vi "Save Symbol.vi"(8 "error in (no error)":errorcluster, 10 "path":path, 11 "proj ref":refnum<vi>) -> (0 "error out":errorcluster, 2 "path out":path, 3 "proj ref out":refnum<vi>)   [LabVIEW 2014, in "lvprj2html.lvlib"]
uses:
  lvprj2html.lvlib
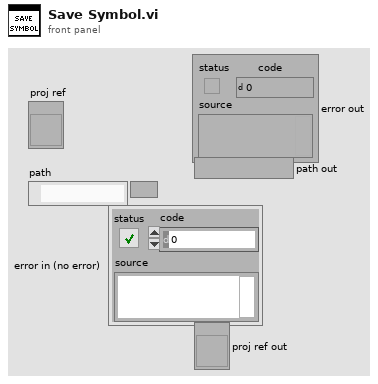
[diagram p1: front panel]
types:
  T1 = typedef "imagedata.ctl" = cluster{"image type":i32, "image depth":i32, "image":u8[], "mask":u8[], "colors":u32[], "Rectangle":cluster{"left":i16, "top":i16, "right":i16, "bottom":i16}}
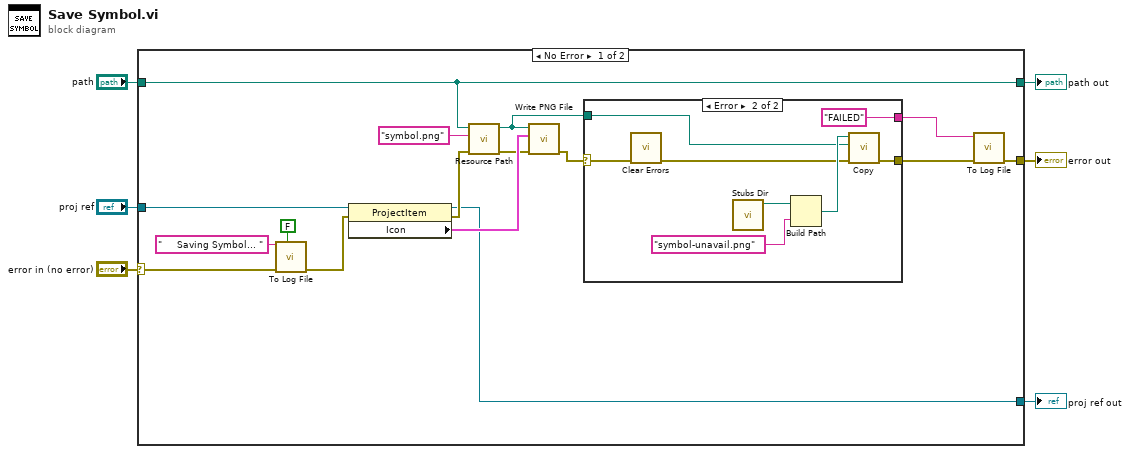
[diagram p0: block diagram]
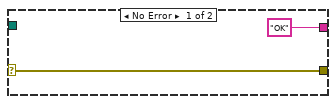
[diagram p2: hidden frame]
diagram:
  n1 = case shown="No Error" "error in (no error)" {
    selector: "error in (no error)" -> [w8 w35]
    tunnel: "proj ref" -> [w21 w33]
    tunnel: [w17 w33] -> w5
    tunnel: "path" -> [w7 w34]
    tunnel: [w9 w35] -> w3
    tunnel: [w7 w34] -> w1
    frame No Error {
      n2 = call "To Log File.vi"("new line"=FALSE, "error in (no error)"=w8, "string"="     Saving Symbol... " ("format string")) -> ("error out"=w14:errorcluster)  [unwired: 8 in]
      n3 = property class="ProjectItem"(reference=w21, error in=w14) -> (reference out=w17:refnum<vi>, error out=w19:errorcluster, "Icon"=w22:T1)
      n4 = call "Resource Path.vi"("error in (no error)"=w19, "resource file name"="symbol.png", "data dir"=w7) -> ("error out"=w18:errorcluster, "path"=w11:path)  [unwired: 7 in]
      n5 = call <vilib>:"Write PNG File.vi"("error in (no error)"=w18, "image data"=w22, "path to PNG file"=w11) -> ("error out"=w10:errorcluster)  [unwired: 7 in, 1 out]
      n6 = case shown="Error" w10 {
        selector: w10 -> [w24 w32]
        tunnel: [w24 w25] -> w12
        tunnel: ["OK" ("string") "FAILED" ("string")] -> w13
        tunnel: w11 -> [_ w27]
        frame No Error {
        }
        frame Error {
          n7 = call <vilib>:"Clear Errors.vi"("error in (no error)"=w32) -> ("error out"=w26:errorcluster)  [unwired: 5 in, 1 out]
          n8 = call "Stubs Dir.vi"() -> ("path"=w29:path)  [unwired: 11 in]
          n9 = Build Path(base path=w29, name or relative path="symbol-unavail.png") -> (appended path=w28:path)
          n10 = call "Copy.vi"("error in (no error)"=w26, "dst"=w27, "src"=w28) -> ("error out"=w25:errorcluster)  [unwired: 8 in]
        }
      }
      n11 = call "To Log File.vi"("error in (no error)"=w12, "string"=w13) -> ("error out"=w9:errorcluster)  [unwired: 9 in]
    }
    frame Error {
    }
  }
  "error out" <- w3
  "path out" <- w1
  "proj ref out" <- w5
